vi "Create Map URL.vi"(4 "Map Format":string(combo)="hybrid", 6 "X":dbl=350.0, 7 "Lat":dbl=51.4062 format="%#.6g", 9 "Y":dbl=570.0, 10 "Zoom":sgl=18.0 format="%#.1g", 11 "Lon":dbl=-1.3070000000000026 format="%#.6g") -> (3 "String":string)   [LabVIEW 2017]
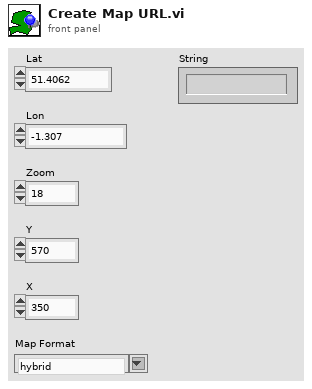
[diagram p1: front panel]
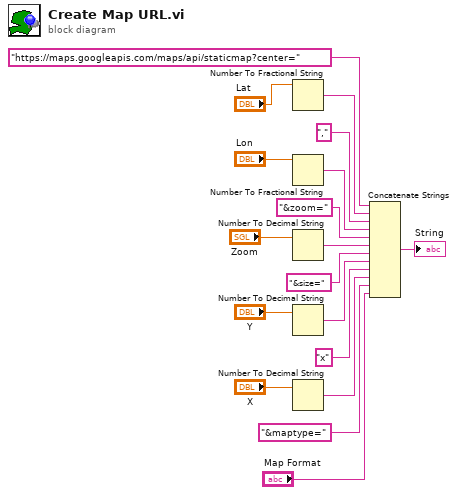
[diagram p0: block diagram]
diagram:
  n1 = Number To Fractional String(number="Lat") -> (F-format string=w16:string)  [unwired: 3 in]
  n2 = Number To Fractional String(number="Lon") -> (F-format string=w18:string)  [unwired: 3 in]
  n3 = Number To Decimal String(number="Zoom") -> (decimal integer string=w7:string)  [unwired: 1 in]
  n4 = Number To Decimal String(number="Y") -> (decimal integer string=w11:string)  [unwired: 1 in]
  n5 = Number To Decimal String(number="X") -> (decimal integer string=w13:string)  [unwired: 1 in]
  n6 = Concatenate Strings("https://maps.googleapis.com/maps/api/staticmap?center=" ("URL"), w16, "," ("string"), w18, "&zoom=", w7, "&size=", w11, "x", w13, "&maptype=", "Map Format") -> (→"String":string)
